vi "Signal_acquisition_v7.vi"() -> ()   [LabVIEW 2015]
uses:
  <vilib>/measure/madcrms.llb/Basic Averaged DC-RMS for 1 Chan.vi
  <vilib>/measure/matone.llb/Extract Single Tone Information 1 Chan.vi
  <vilib>/express/express arith-compare/Formula/XNode/ExpressFormulaBlockNode.xnode
  <vilib>/measure/NI_MAPro.lvlib
panel:
  in  "timeout ms":i32=2000
  in  "timeout ms\n (2000)":i32=2000
  in  "timeout ms\n (2000) 2":i32=2000
  in  "Delay\n (# Samples)":i32 max=16348
  in  "Trigger Level \n(0 mV)":i32
  out "DC value 2":dbl format="%0.2p"
  out "detected \nfrequency 2":dbl format="%.2p"
  out "Ieration\nnumber":i32
  out "millisecond \ntimer value":u32
  out "millisecond \nbegin timer":u32
  out "millisecond \nfinal timer":u32
  in  "Tab Control":T1(tab)
  out "Voltage Gain / Frequency":cluster{i32, dbl}[](graph)
  out "Cutoff Freqs (Hz)":i32[](array[numeric])
  in  "MEASURE AMPLITUD":bool
  out "Acquisition\ntime complete":u32
  out "MEASURED \namplitud":dbl format="%.2p"
  out "RESULT \nin amplittude":dbl
  out "FRECUENCY \nEND":i32
  out "detected \nphase (deg)":dbl format="%.2p"
  out "detected \nfrequency":dbl format="%.2p"
  in  "Filename":path=path "test.xlsx"
  in  "Trigger Mode":string(combo)="CH1_NE"
  in  "input":u16=1
  in  "Pause \nfor buffer (ms)":u32=100
  out "error out":errorcluster
  in  "VOLTS":dbl=0.1
  in  "FREQ END":i32=70000
  in  "FREQ START":i32=10000
  in  "number \nof intervals":i32=60
  in  "IP address":string="192.168.0.10"
  in  "error in":errorcluster
  in  "Automatic decimation":bool=TRUE
  in  "Decimation":u16(ring)=8 items=["65536"=65535, "8192"=8192, "1024"=1024, "64"=64, "8"=8, "1"=1]
  out "REAL TIME MEASUREMENT":dbl[](graph)
  in  "FREQ START 5":i32
  in  "number of intervals  3":i32
  in  "number of intervals  2":i32
  # "FREQUENCY SWEEP"
  # "FREQUENCY SWEEP"
  # "Settings parameters"
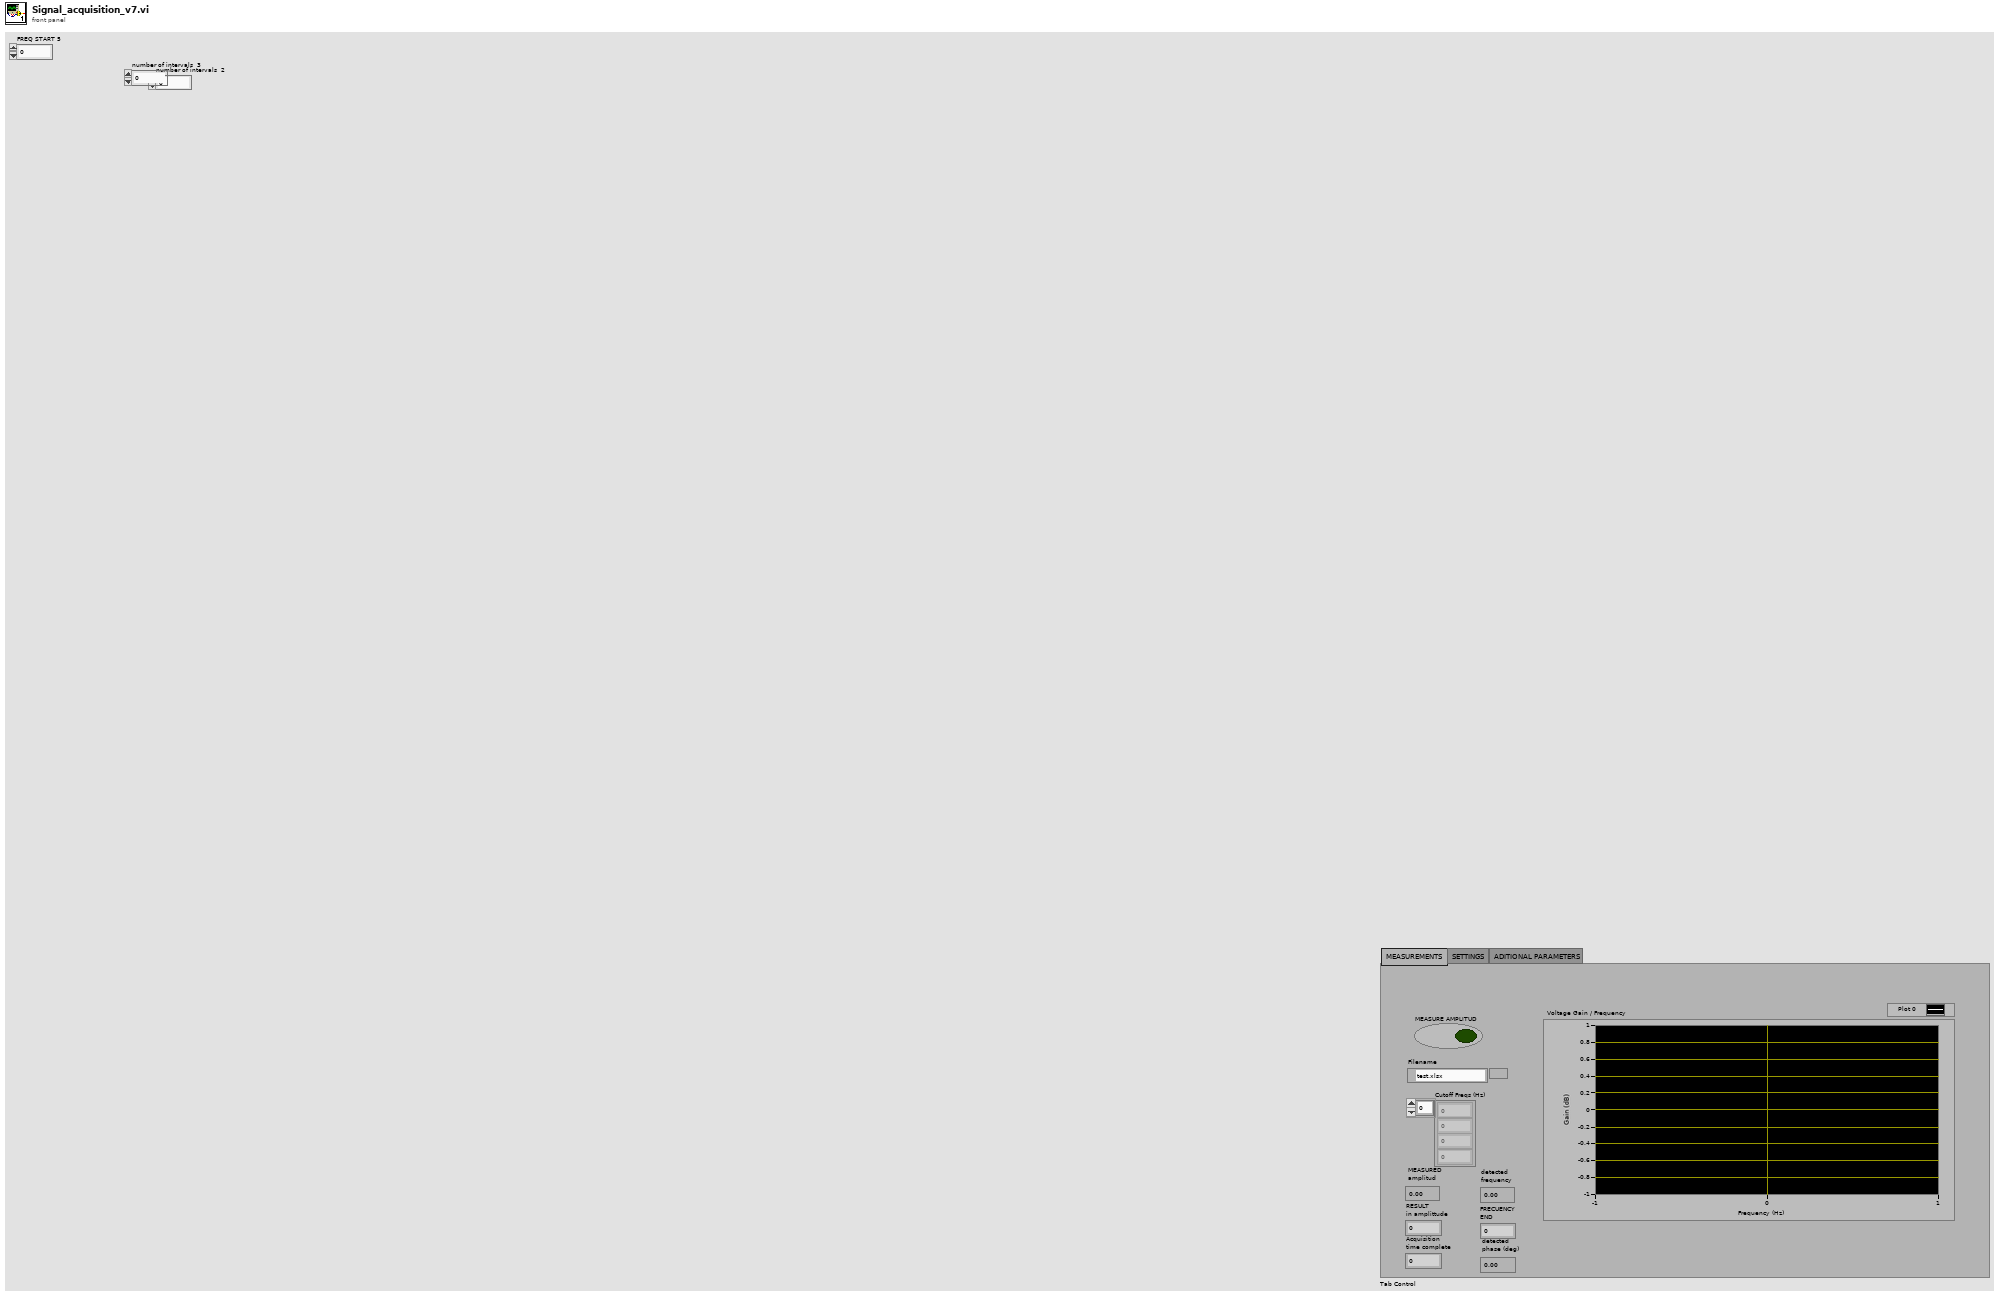
[diagram p1: front panel]
types:
  T1 = enum32{"MEASUREMENTS ", "SETTINGS", "ADITIONAL PARAMETERS"}
  T2 = enum32{"none", "input signal", "detected signal", "residual signal"}
  T3 = enum16{"Standard", "Buffered", "CRLF", "Immediate"}
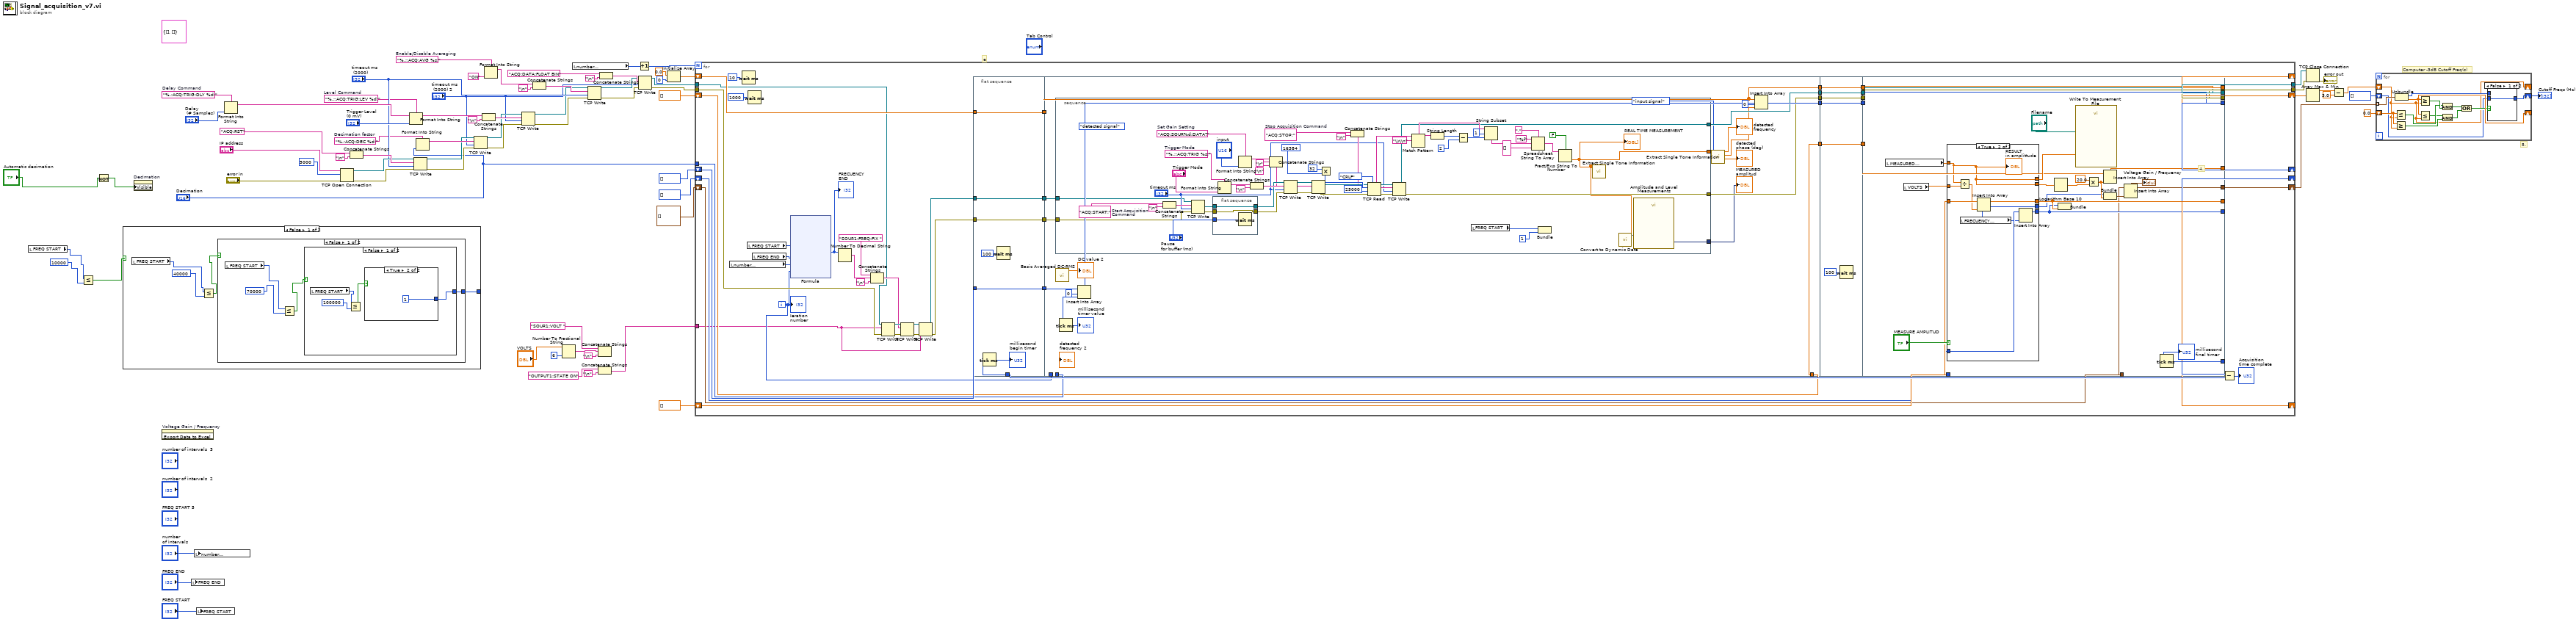
[diagram p0: block diagram]
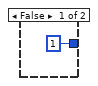
[diagram p2: hidden frame]
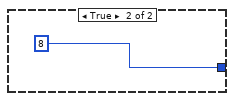
[diagram p3: hidden frame]
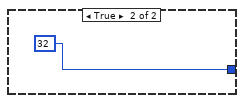
[diagram p4: hidden frame]
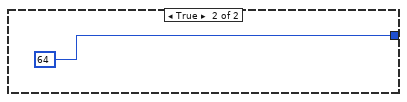
[diagram p5: hidden frame]
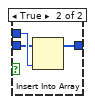
[diagram p6: hidden frame]
diagram:
  (unwired) cluster{dbl[], dbl[]} {[], []} ("FRECUENCY SWEEP")
  w42 = "%.;:ACQ:AVG %s;"  # Enable/Disable Averaging
  w50 = "%.;ACQ:DEC %d;"  # Decimation factor
  w51 = "%.;ACQ:TRIG:DLY %d;"  # Delay Command
  w52 = "%.;:ACQ:TRIG:LEV %d;"  # Level Command
  # "5."
  # "Computer -3dB Cutoff Freq(s)"
  # "e"
  n1 = local read "FREQ START"() -> (w6:i32)
  n2 = Less Or Equal?(x=w6, y=10000) -> (x <= y?=w4:bool)
  n3 = Not(x="Automatic decimation") -> (.not. x?=w1:bool)
  n4 = case shown="False" w4 {
    tunnel: [w80 64] -> _
    frame False {
      n5 = local read "FREQ START"() -> (w79:i32)
      n6 = Less Or Equal?(x=w79, y=40000) -> (x <= y?=w77:bool)
      n7 = case shown="False" w77 {
        tunnel: [w84 32] -> w80
        frame False {
          n8 = local read "FREQ START"() -> (w82:i32)
          n9 = Less Or Equal?(x=w82, y=70000) -> (x <= y?=w81:bool)
          n10 = case shown="False" w81 {
            tunnel: [w88 8] -> w84
            frame False {
              n11 = local read "FREQ START"() -> (w87:i32)
              n12 = Less Or Equal?(x=w87, y=100000) -> (x <= y?=w85:bool)
              n13 = case shown="True" w85 {
                tunnel: [1 1] -> w88
                frame False {
                }
                frame True {
                }
              }
            }
            frame True {
            }
          }
        }
        frame True {
        }
      }
    }
    frame True {
    }
  }
  n14 = property on="Decimation" class="Ring (strict)"("Visible"=w1) -> ()  [unwired: 2 in, 2 out]
  n15 = invoke on="Voltage Gain / Frequency" class="XYGraph (strict)" method="Export Data to Excel"() -> ()  [unwired: 3 in, 3 out]
  n16 = local write "FREQ END"("FREQ END") -> ()
  n17 = local write "number \nof intervals"("number \nof intervals") -> ()
  n18 = local write "FREQ START"("FREQ START") -> ()
  n19 = Format Into String(format string=w51, "Delay\n (# Samples)") -> (resulting string=w70:string)  [unwired: 2 in, 1 out]
  n20 = TCP Open Connection(address="IP address", remote port or service name=u16 5000, error in (no error)="error in") -> (connection ID=w64:refnum<k5>, error out=w63:errorcluster)  [unwired: 2 in]
  n21 = Concatenate Strings("ACQ:RST" ("SCPI Message"), "\n") -> (w66:string)
  n22 = Format Into String(format string=w52, initial string=w70, "Trigger Level \n(0 mV)") -> (resulting string=w67:string)  [unwired: 1 in, 1 out]
  n23 = TCP Write(connection ID=w64, data in=w66, error in (no error)=w63, 9:"timeout ms\n (2000)") -> (connection ID out=w48:refnum<k5>, error out=w47:errorcluster)  [unwired: 1 out]
  n24 = Format Into String(format string=w50, "Decimation") -> (resulting string=w49:string)  [unwired: 2 in, 1 out]
  n25 = TCP Write(connection ID=w48, data in=w49, error in (no error)=w47, 9:"timeout ms\n (2000) 2") -> (connection ID out=w46:refnum<k5>, error out=w45:errorcluster)  [unwired: 1 out]
  n26 = Concatenate Strings(w67, "\n") -> (w61:string)
  n27 = Format Into String(format string=w42, "ON") -> (resulting string=w73:string)  [unwired: 2 in, 1 out]
  n28 = TCP Write(connection ID=w46, data in=w61, error in (no error)=w45, 9:"timeout ms\n (2000) 2") -> (connection ID out=w44:refnum<k5>, error out=w43:errorcluster)  [unwired: 1 out]
  n29 = Concatenate Strings(w73, "\n") -> (w62:string)
  n30 = Number To Fractional String(number="VOLTS", precision (6)=i16 6) -> (F-format string=w13:string)  [unwired: 2 in]
  n31 = local read "number \nof intervals"() -> (w29:i32)
  n32 = TCP Write(connection ID=w44, data in=w62, error in (no error)=w43, 9:"timeout ms\n (2000)") -> (connection ID out=w40:refnum<k5>, error out=w39:errorcluster)  [unwired: 1 out]
  n33 = Concatenate Strings("SOUR1:VOLT " ("SCPI Message"), w13, "\n") -> ()  [unwired: 1 out]
  n34 = Concatenate Strings("OUTPUT1:STATE ON" ("SCPI Message"), "\n") -> (w7:string)
  n35 = Concatenate Strings("ACQ:DATA:FLOAT BIN" ("SCPI Message"), "\n") -> (w58:string)
  n36 = Increment(x=w29) -> (x+1=w28:i32)
  n37 = TCP Write(connection ID=w40, data in=w58, error in (no error)=w39, 9:"timeout ms\n (2000) 2") -> (connection ID out=w37:refnum<k5>, error out=w36:errorcluster)  [unwired: 1 out]
  n38 = Initialize Array(0.0 ("element"), 0 ("dimension size")) -> (w32:dbl[])
  n39 = for {
    N: w28 -> [_]
    tunnel: w37 -> [w125]
    tunnel: [w143] -> w57
    tunnel: [w142] -> w56
    tunnel: w36 -> [w122]
    shift-right: [w145] -> _
    shift-left: u32[] [] -> [w144]
    tunnel: "Decimation" -> [w135]
    shift-right: [w133] -> _
    shift-left: w32 -> [w131]
    shift-right: [w118] -> _
    shift-left: dbl[] [] -> [w119]
    shift-right: [w114] -> _
    shift-left: i32[] [] -> [w113]
    shift-right: [w109] -> w17
    shift-left: dbl[] [] -> [w108]
    shift-right: [w107] -> w16
    shift-left: cluster{"FRECUENCY END":i32, dbl}[] [] -> [w106]
    tunnel: w7 -> [w94]
    i -> [w95]
    n40 = local read "number \nof intervals"() -> (w115:i32)
    n41 = Wait (ms)(milliseconds to wait=u32 10) -> ()  [unwired: 1 out]
    n42 = local read "FREQ START"() -> (w116:i32)
    n43 = Wait (ms)(milliseconds to wait=u32 1000) -> ()  [unwired: 1 out]
    n44 = local read "FREQ END"() -> (w117:i32)
    n45 = xnode "Formula"("Fin"=w116, "Fend"=w117, "Ninter"=w115, "i"=w95) -> ("Result"=w110:i32)  [unwired: 1 in, 1 out]
    "FRECUENCY \nEND" <- w110
    n46 = Number To Decimal String(number=w110) -> (decimal integer string=w120:string)  [unwired: 1 in]
    n47 = Concatenate Strings("SOUR1:FREQ:FIX " ("SCPI Message"), w120, "\n") -> (w126:string)
    n48 = TCP Write(connection ID=w125, data in=w94, error in (no error)=w122) -> (connection ID out=w129:refnum<k5>, error out=w128:errorcluster)  [unwired: 1 in, 1 out]
    n49 = TCP Write(connection ID=w129, data in=w126, error in (no error)=w128) -> (connection ID out=w112:refnum<k5>, error out=w111:errorcluster)  [unwired: 1 in, 1 out]
    n50 = TCP Write(connection ID=w112, data in=w94, error in (no error)=w111) -> (connection ID out=w124:refnum<k5>, error out=w123:errorcluster)  [unwired: 1 in, 1 out]
    n51 = flat-sequence {
      tunnel: w144 -> [w163]
      tunnel: w123 -> [w164]
      tunnel: w124 -> [w165]
      tunnel: [w165] -> w141
      tunnel: [w164] -> w140
      tunnel: [w163] -> w139
      tunnel: [w162] -> w137
      tunnel: [w161] -> w132
      tunnel: w131 -> [w161]
      tunnel: [w179] -> w105
      tunnel: [w177] -> w103
      tunnel: [w176] -> w101
      tunnel: w141 -> [w183]
      tunnel: w140 -> [w182]
      tunnel: w139 -> [w178]
      tunnel: w135 -> [_]
      tunnel: [w172] -> w99
      tunnel: w95 -> [_]
      tunnel: w132 -> [w172]
      tunnel: w108 -> [w168]
      tunnel: [w168] -> w97
      tunnel: w105 -> [w248]
      tunnel: [w248] -> w104
      tunnel: w103 -> [w247]
      tunnel: [w247] -> w102
      tunnel: w101 -> [w246]
      tunnel: [w246] -> w100
      tunnel: w99 -> [w245]
      tunnel: [w245] -> w98
      tunnel: w97 -> [w244]
      tunnel: [w244] -> w96
      tunnel: [w270] -> w142
      tunnel: [w271] -> w143
      tunnel: [w272] -> w145
      tunnel: w104 -> [w272]
      tunnel: w102 -> [w271]
      tunnel: w100 -> [w270]
      tunnel: [w269] -> w138
      tunnel: w98 -> [w268]
      tunnel: [w268] -> w133
      tunnel: w119 -> [w264]
      tunnel: [w262] -> w118
      tunnel: [w261] -> w114
      tunnel: w113 -> [w263]
      tunnel: [w256] -> w109
      tunnel: w96 -> [w255]
      tunnel: [w253] -> w107
      tunnel: w106 -> [w252]
      frame #0 {
        n52 = Tick Count (ms)() -> (millisecond timer value=w162:u32)
        "millisecond \nbegin timer" <- w162
        n53 = Wait (ms)(milliseconds to wait=u32 100) -> ()  [unwired: 1 out]
      }
      frame #1 {
        n54 = stacked-sequence {
          tunnel: w183 -> [w189]
          tunnel: w182 -> [w192]
          tunnel: [w190] -> w177
          tunnel: [w191] -> w176
          tunnel: [w186] -> w170
          tunnel: [w184] -> w166
          frame #0 {
            w199 = "ACQ:STOP;"  # Stop Acquisition Command
            (unwired) T2."detected signal" ("export mode")
            w209 = "ACQ:SOUR%d:DATA?"  # Set Gain Setting
            w236 = "%.;:ACQ:TRIG %s;"  # Trigger Mode
            w238 = "ACQ:START;"  # Start Acquisition Command
            n55 = Concatenate Strings(w238, "\n") -> (w239:string)
            n56 = TCP Write(connection ID=w189, data in=w239, error in (no error)=w192, 9:"timeout ms") -> (connection ID out=w213:refnum<k5>, error out=w212:errorcluster)  [unwired: 1 out]
            n57 = flat-sequence {
              tunnel: "Pause \nfor buffer (ms)" -> [w242]
              tunnel: [w241] -> w211
              tunnel: [w240] -> w210
              tunnel: w213 -> [w241]
              tunnel: w212 -> [w240]
              frame #0 {
                n58 = Wait (ms)(milliseconds to wait=w242) -> ()  [unwired: 1 out]
              }
            }
            n59 = Format Into String(format string=w236, "Trigger Mode") -> (resulting string=w233:string)  [unwired: 2 in, 1 out]
            n60 = Format Into String(format string=w209, "input") -> (resulting string=w207:string)  [unwired: 2 in, 1 out]
            n61 = Concatenate Strings(w233, "\n") -> (w234:string)
            n62 = Concatenate Strings(w207, "\r", "\n") -> (w206:string)
            n63 = TCP Write(connection ID=w211, data in=w234, error in (no error)=w210, 9:"timeout ms") -> (connection ID out=w204:refnum<k5>, error out=w203:errorcluster)  [unwired: 1 out]
            n64 = TCP Write(connection ID=w204, data in=w206, error in (no error)=w203) -> (connection ID out=w205:refnum<k5>, error out=w202:errorcluster)  [unwired: 1 in, 1 out]
            n65 = Multiply(x=32, y=16384 ("bytes to read")) -> (x*y=w214:i32)
            n66 = Concatenate Strings(w199, "\n") -> (w197:string)
            n67 = TCP Read(connection ID=w205, bytes to read=w214, error in (no error)=w202, 7:T3."CRLF" ("mode (standard)"), 9:25000 ("timeout ms (25000)")) -> (connection ID out=w200:refnum<k5>, data out=w215:string, error out=w196:errorcluster)
            n68 = TCP Write(connection ID=w200, data in=w197, error in (no error)=w196, 9:"timeout ms") -> (connection ID out=w190:refnum<k5>, error out=w191:errorcluster)  [unwired: 1 out]
            n69 = Match Pattern(string=w215, regular expression="\\r\\n") -> (before substring=w221:string)  [unwired: 1 in, 3 out]
            n70 = String Length(string=w221) -> (length=w224:i32)
            n71 = Subtract(x=w224, y=2) -> (x-y=w225:i32)
            n72 = local read "FREQ START"() -> (w188:i32)
            n73 = String Subset(string=w221, offset (0)=1, length (rest)=w225) -> (substring=w222:string)
            n74 = Spreadsheet String To Array(delimiter (Tab)=",", format string="%f", spreadsheet string=w222, array type (2D Dbl)=string[] [] ("Array")) -> (array=w228:string[])
            n75 = Bundle("FREQ START"=w188, 1) -> ()  [unwired: 1 in, 1 out]
            n76 = Fract/Exp String To Number(use system decimal point (T)=FALSE, string=w228) -> (number=w186:dbl[])  [unwired: 3 out]
            "REAL TIME MEASUREMENT" <- w186
            n77 = call-poly <vilib>:"Extract Single Tone Information.vi"("time signal in"=w186) -> ()  [unwired: 5 in, 6 out]
            n78 = call "Convert to Dynamic Data"("Array"=w186) -> ("Dynamic Data Type"=w185:dynamicdata)  [unwired: 3 in]
            n79 = call "Amplitude and Level Measurements"("Signals"=w185) -> ("Peak to Peak"=w184:dynamicdata)  [unwired: 13 in, 1 out]
          }
        }
        "MEASURED \namplitud" <- w166
        n80 = call-poly <vilib>:"Basic Averaged DC-RMS.vi"() -> ("DC value"=→"DC value 2":dbl)  [unwired: 8 in, 3 out]
        n81 = Tick Count (ms)() -> (millisecond timer value=w180:u32)
        "millisecond \ntimer value" <- w180
        n82 = Insert Into Array(array=w178, index=0, new element=w180) -> (w179:u32[])
        n83 = call-poly <vilib>:"Extract Single Tone Information.vi"("export mode"=T2."input signal", "time signal in"=w170) -> ("detected phase (deg)"=→"detected \nphase (deg)":dbl, "detected amplitude"=w169:dbl, "detected frequency"=→"detected \nfrequency":dbl)  [unwired: 4 in, 3 out]
        n84 = Insert Into Array(array=w172, index=0, new element=w169) -> ()  [unwired: 1 out]
      }
      frame #2 {
        n85 = Wait (ms)(milliseconds to wait=u32 100) -> ()  [unwired: 1 out]
      }
      frame #3 {
        # "4."
        n86 = local read "MEASURED \namplitud"() -> (w267:dbl)
        n87 = local read "VOLTS"() -> (w250:dbl)
        n88 = case shown="True" "MEASURE AMPLITUD" {
          tunnel: w267 -> [_ w277]
          tunnel: [w273 w277] -> w265
          tunnel: w264 -> [w275 w283]
          tunnel: [w275 w282] -> w262
          tunnel: [w274 w281] -> w261
          tunnel: w263 -> [w274 w280]
          tunnel: [_ w277] -> w251
          tunnel: [_ w279] -> w254
          tunnel: w250 -> [w273 w278]
          frame False {
          }
          frame True {
            n89 = Divide(x=w277, y=w278) -> (x/y=w276:dbl)
            n90 = local read "FRECUENCY \nEND"() -> (w279:i32)
            n91 = Insert Into Array(array=w283, new element=w276) -> (w282:dbl[])  [unwired: 1 in]
            n92 = Insert Into Array(array=w280, new element=w279) -> (w281:i32[])  [unwired: 1 in]
            "RESULT \nin amplittude" <- w277
          }
        }
        n93 = Logarithm Base 10(1:w251) -> (0:w258:dbl)
        n94 = Bundle(w261, w262) -> ()  [unwired: 1 in, 1 out]
        n95 = call "Write To Measurement File"("Signals"=w265, "Filename"="Filename") -> ()  [unwired: 15 in, 3 out]
        n96 = Multiply(x=20.0, y=w258) -> (x*y=w257:dbl)
        n97 = Insert Into Array(array=w255, new element=w257) -> (w256:dbl[])  [unwired: 1 in]
        n98 = Bundle("FRECUENCY \nEND"=w254, w257) -> (w260:cluster{"FRECUENCY \nEND":i32, dbl})  [unwired: 1 in]
        n99 = Insert Into Array(array=w252, new element=w260) -> (w253:cluster{"FRECUENCY END":i32, dbl}[])  [unwired: 1 in]
        "Voltage Gain / Frequency" <- w253
        n100 = Tick Count (ms)() -> (millisecond timer value=w269:u32)
        "millisecond \nfinal timer" <- w269
      }
    }
    n101 = Subtract(x=w138, y=w137) -> (x-y=→"Acquisition\ntime complete":u32)
    "Ieration\nnumber" <- w95
  }
  n102 = TCP Close Connection(connection ID=w57, error in (no error)=w56) -> (error out=→"error out":errorcluster)  [unwired: 1 in, 1 out]
  n103 = Array Max & Min(array=w17) -> (max value=w18:dbl)  [unwired: 3 out]
  n104 = Subtract(x=w18, y=3.0) -> (x-y=w19:dbl)
  n105 = for {
    tunnel: w16 -> [w297] mode=indexing
    shift-right: [w291] -> _
    shift-left: 0.0 -> [w292]
    shift-right: [w285] -> w21
    shift-left: i32[] [] -> [w286]
    shift-right: [w284] -> _
    shift-left: w19 -> [w284]
    n106 = Less Or Equal?(x=w292, y=w284) -> (x <= y?=w295:bool)
    n107 = Greater Or Equal?(x=w292, y=w284) -> (x >= y?=w293:bool)
    n108 = Unbundle(w297) -> ("FRECUENCY END"=w287:i32, w291:dbl)
    n109 = Greater Or Equal?(x=w291, y=w284) -> (x >= y?=w296:bool)
    n110 = Less Or Equal?(x=w291, y=w284) -> (x <= y?=w294:bool)
    n111 = And(x=w295, y=w296) -> (x .and. y?=w289:bool)
    n112 = And(x=w294, y=w293) -> (x .and. y?=w290:bool)
    n113 = Or(x=w289, y=w290) -> (x .or. y?=w288:bool)
    n114 = case shown="False" w288 {
      tunnel: w287 -> [_ w301]
      tunnel: w286 -> [w298 w300]
      tunnel: [w298 w299] -> w285
      frame False {
      }
      frame True {
        n115 = Insert Into Array(array=w300, new element=w301) -> (w299:i32[])  [unwired: 1 in]
      }
    }
  }
  "Cutoff Freqs (Hz)" <- w21
